vi "TLB Native Dynamic Events ver 0.06.vi"() -> ()   [LabVIEW 2018]
uses:
  Labview Training Phase 2/Enum Controls/States for Action Engine.ctl
  Type def/TLB event states.ctl
  Type def/TLB MHL States.ctl
  <vilib>/Studica/Studica Toolkit/Background/I2C Channel.ctl
  <vilib>/Studica/Studica Toolkit/NavX/NavX.lvlib
  <vilib>/myRIO/Common/Instrument Driver Framework/myRIO v1.0/AI/typedefs/AI Channels Enum.ctl
  <vilib>/myRIO/Common/Instrument Driver Framework/myRIO v1.0/AI/typedefs/AI Channels List.ctl
  <vilib>/Studica/Studica Toolkit/Background/Mxp Selection.ctl
  <vilib>/ptbypt/NI_PtbyPt.lvlib
  Type def/Type def.ctl
  Type def/Motor Control Cluster.ctl
  <vilib>/Studica/Studica Blackhawk/Blackhawk.lvlib
  <vilib>/vision/driver/NI_Vision_Acquisition_Software.lvlib
  <vilib>/userdefined/High Color/IMAQdx.ctl
  <vilib>/vision/driver/IMAQdx.llb/IMAQdx Buffer Number Mode.ctl
  <vilib>/vision/driver/IMAQdx.llb/IMAQdx Acquisition Mode.ctl
panel:
  in  "Camera ENA":bool
  out "Right IR Sensor":dbl
  out "Left IR Sensor":dbl
  out "CM":fxp<+,64,16>
  out "Ultrasonic sensor":dbl format="%0.2f"
  in  "Servo Angle":u8(slide) scale=0.0..180.0
  in  "On/Off":bool
  out "Blackhawk error":errorcluster
  out "Value Read":bool
  out "Image Processing error":errorcluster
  out "Image Out":T1(plugin-control)
  out "element":T2
  out "Action Queue Items":i32
  out "State Logic Queue Items":i32
  out "Action Queues items":string[](array[string])=["Hardware reset", "Software reset", ""]
  out "State logic":T3=enum."Task 2"
  out "Action State":string
  in  "Tasks Selector":string(combo)="Task 2"
  out "Distance":T4
  in  "xTargetSpeed":dbl
  in  "yTargetSpeed":dbl
  in  "wTargetSpeed":dbl
  out "Speed":T5
  out "Yaw":dbl
  out "NavX Info Out":T7
  out "LinearAcceleration":T8
  out "Displacement":T9
  out "YRPHfH":T10
  out "Object detected":bool
  in  "NavX Zero Yaw":bool
  in  "Return to IDLE":bool
  in  "Reset Encoder 0":bool
  in  "Stop Queue":bool
  in  "Start Task":bool
  # "Sensor data"
  # "Blackhawk status"
  # "Camera Status Loop"
  # "TLB FRAMEWORK STATUS"
  # "Test Programme written by Calvin Loke    Dated: 28 Aug 2019\nTest Programme revised by Dr Alex See   Dated 30 Aug 2019\n\nProgramme version:   TLB Native Dynamic Events ver 0.04b.vi"
  # "Sequence of Actions"
  # "Continuous (Repeated)"
  # "System Health Status Update"
  # "Motor Control Loop"
  # "NAVX Control Loop"
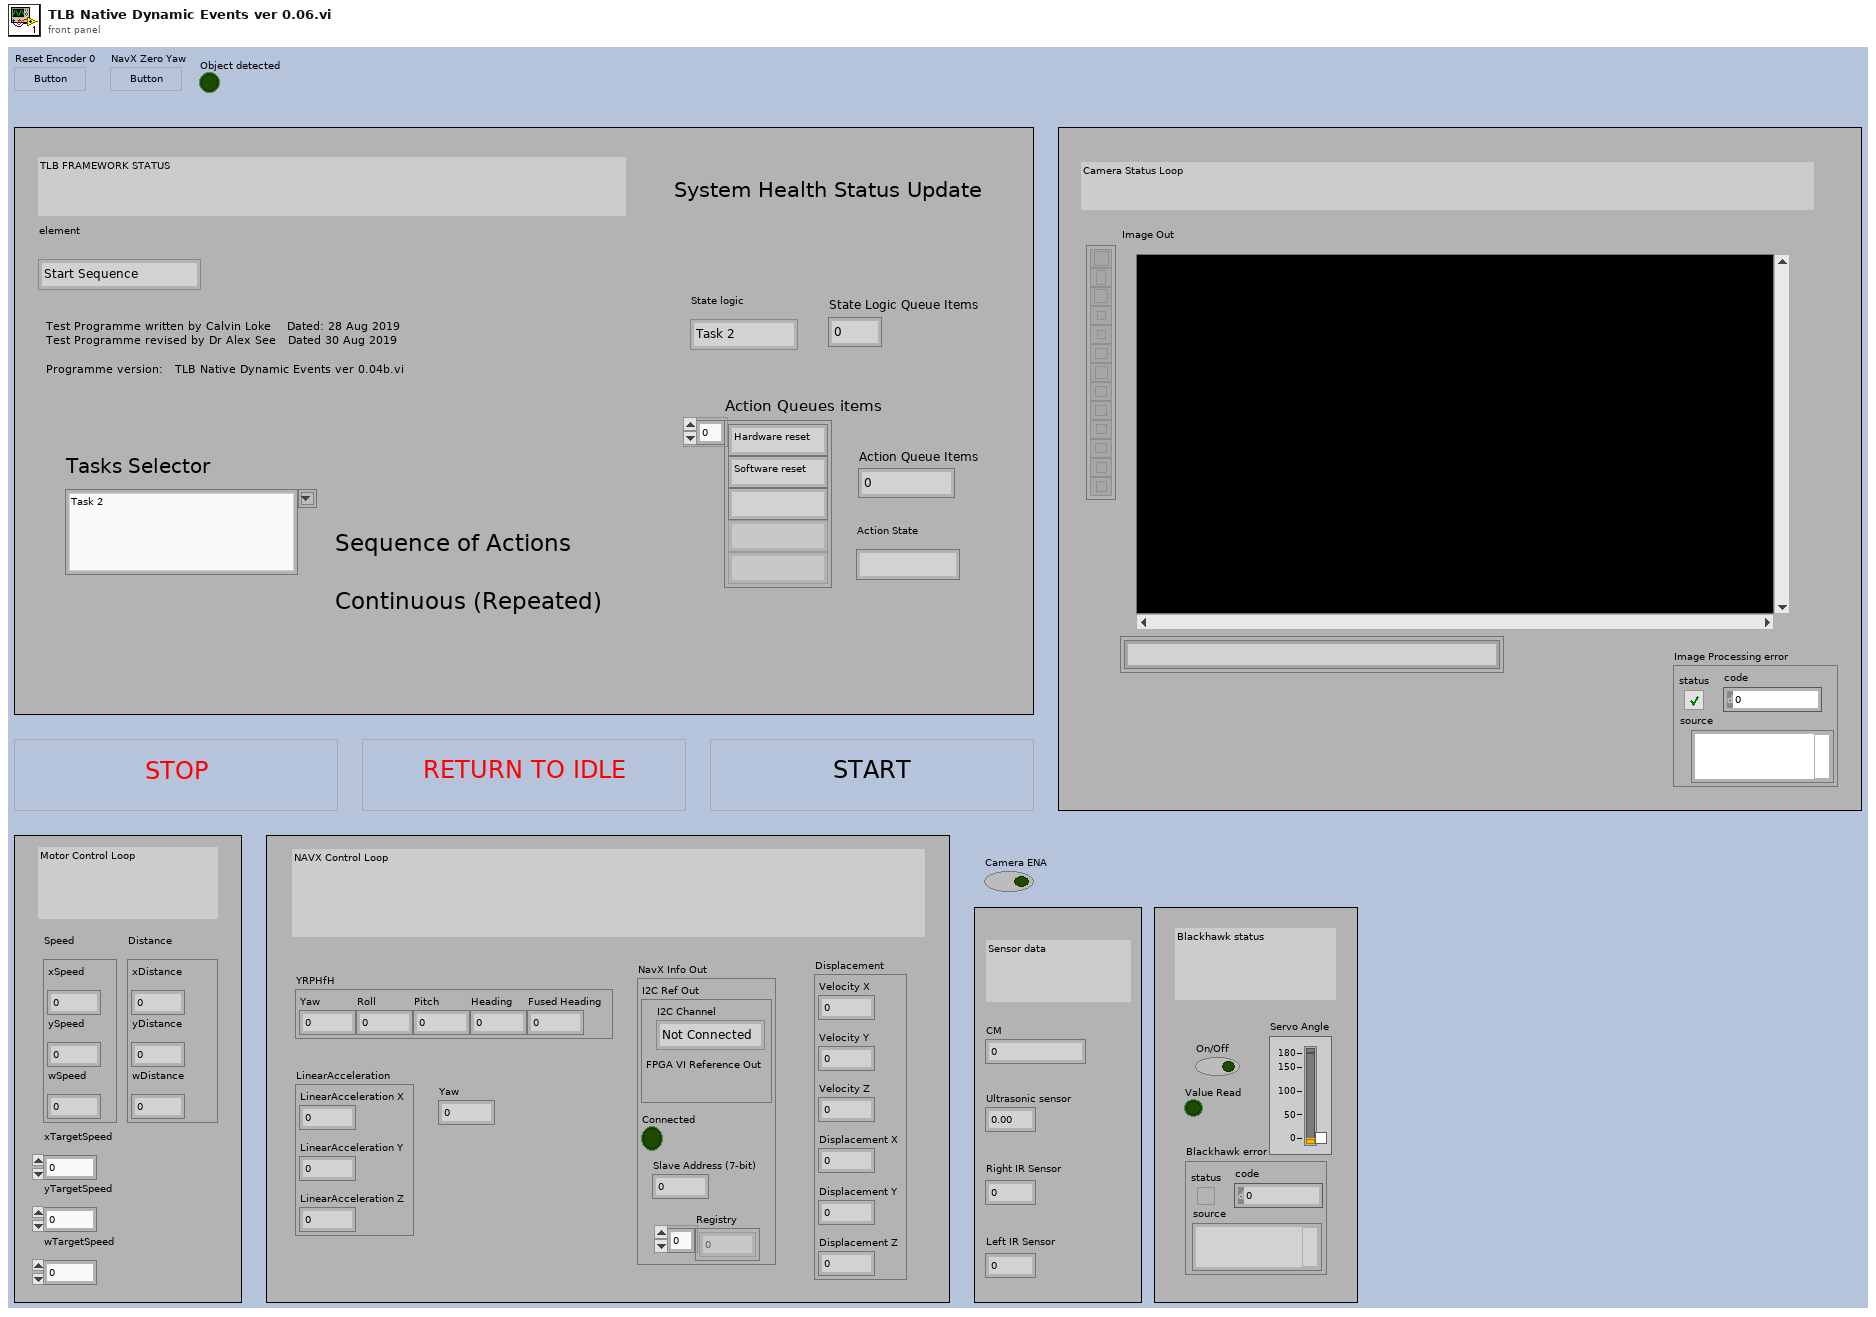
[diagram p1: front panel]
types:
  T1 = typedef "IMAQ Image.ctl" = refnum<image>
  T2 = typedef "TLB event states.ctl" = enum16{"Start Sequence", "Exit", "Start Task 1", "Start Task 2", "Start Task 3", "Start Task 4", "Camera vision", "Wall follow mode", "Idle", "Start Drive Straight"}
  T3 = typedef "TLB MHL States.ctl" = enum16{"None", "Startup", "Idle", "Processing", "Shutdown", "Reset", "Task 1", "Task 2", "Task 3", "Task 4", "Task 4a", "Task 4b", "Task 4c", "Task 4d", "Task 4e", "Task 4f", "Task 4g", "Task 4h", "Acquire image", "Wall follow mode", "Autodrive", "Autodrive a"}
  T4 = cluster{"xDistance":dbl, "yDistance":dbl, "wDistance":dbl}
  T5 = cluster{"xSpeed":dbl, "ySpeed":dbl, "wSpeed":dbl}
  T6 = typedef "I2C Channel.ctl" = enum16{"Not Connected", "A", "B"}
  T7 = cluster{"I2C Ref Out":cluster{"I2C Channel":T6, "FPGA VI Reference Out":refnum<k20>}, "Connected":bool, "Slave Address (7-bit)":u8, "Registry":u8[]}
  T8 = cluster{"LinearAcceleration X":dbl, "LinearAcceleration Y":dbl, "LinearAcceleration Z":dbl}
  T9 = cluster{"Velocity X":dbl, "Velocity Y":dbl, "Velocity Z":dbl, "Displacement X":dbl, "Displacement Y":dbl, "Displacement Z":dbl}
  T10 = cluster{"Yaw":dbl, "Roll":dbl, "Pitch":dbl, "Heading":dbl, "Fused Heading":dbl}
  T11 = typedef "States for Action Engine.ctl" = enum16{"Initialize", "Write", "Read"}
  T12 = typedef "NI_Vision_Acquisition_Software.lvlib/IMAQdx Acquisition Mode.ctl" = enum32{"One Shot", "Continuous"}
  T13 = typedef "IMAQdx.ctl" = refnum<k21>
  T14 = typedef "Motor Control Cluster.ctl" = cluster{"Vx":dbl, "Vy":dbl, "Vw":dbl}
  T15 = typedef "Type def.ctl" = cluster{"Front Ultrasonic Obstruct":bool, "Left Ultrasonic Obstruct":bool, "Right Ultrasonic Obstruct ":bool}
  T16 = typedef "NI_Vision_Acquisition_Software.lvlib/IMAQdx Buffer Number Mode.ctl" = enum32{"Next", "Last", "Buffer Number", "Every", "Last New"}
  T17 = typedef "Mxp Selection.ctl" = enum16{"MXP A", "MXP B"}
  T18 = typedef "TLB event states.ctl" = enum16{"Start Sequence", "Exit", "Start Task 1", "Start Task 2", "Start Task 3", "Start Task 4", "RT Camera tracking", "Wall follow mode", "Idle"}
  T19 = cluster{"I2C Channel":T6, "FPGA VI Reference Out":refnum<k20>}
  T20 = typedef "AI Channels List.ctl" = T21[]
  T21 = typedef "AI Channels Enum.ctl" = enum16{"Not Connected", "AudioIn/Left", "AudioIn/Right", "C/AI0", "C/AI1", "A/AI0", "A/AI1", "A/AI2", "A/AI3", "A/AI4", "A/AI5", "A/AI6", "A/AI7", "B/AI0", "B/AI1", "B/AI2", "B/AI3", "B/AI4", "B/AI5", "B/AI6", "B/AI7", "AI/AI0", "AI/AI1", "AI/AI2", "AI/AI3", "A/AI0 (DIFF)", "A/AI1 (DIFF)", "A/AI2 (DIFF)", "A/AI3 (DIFF)", "B/AI0 (DIFF)", "B/AI1 (DIFF)", "B/AI2 (DIFF)", "B/AI3 (DIFF)"}
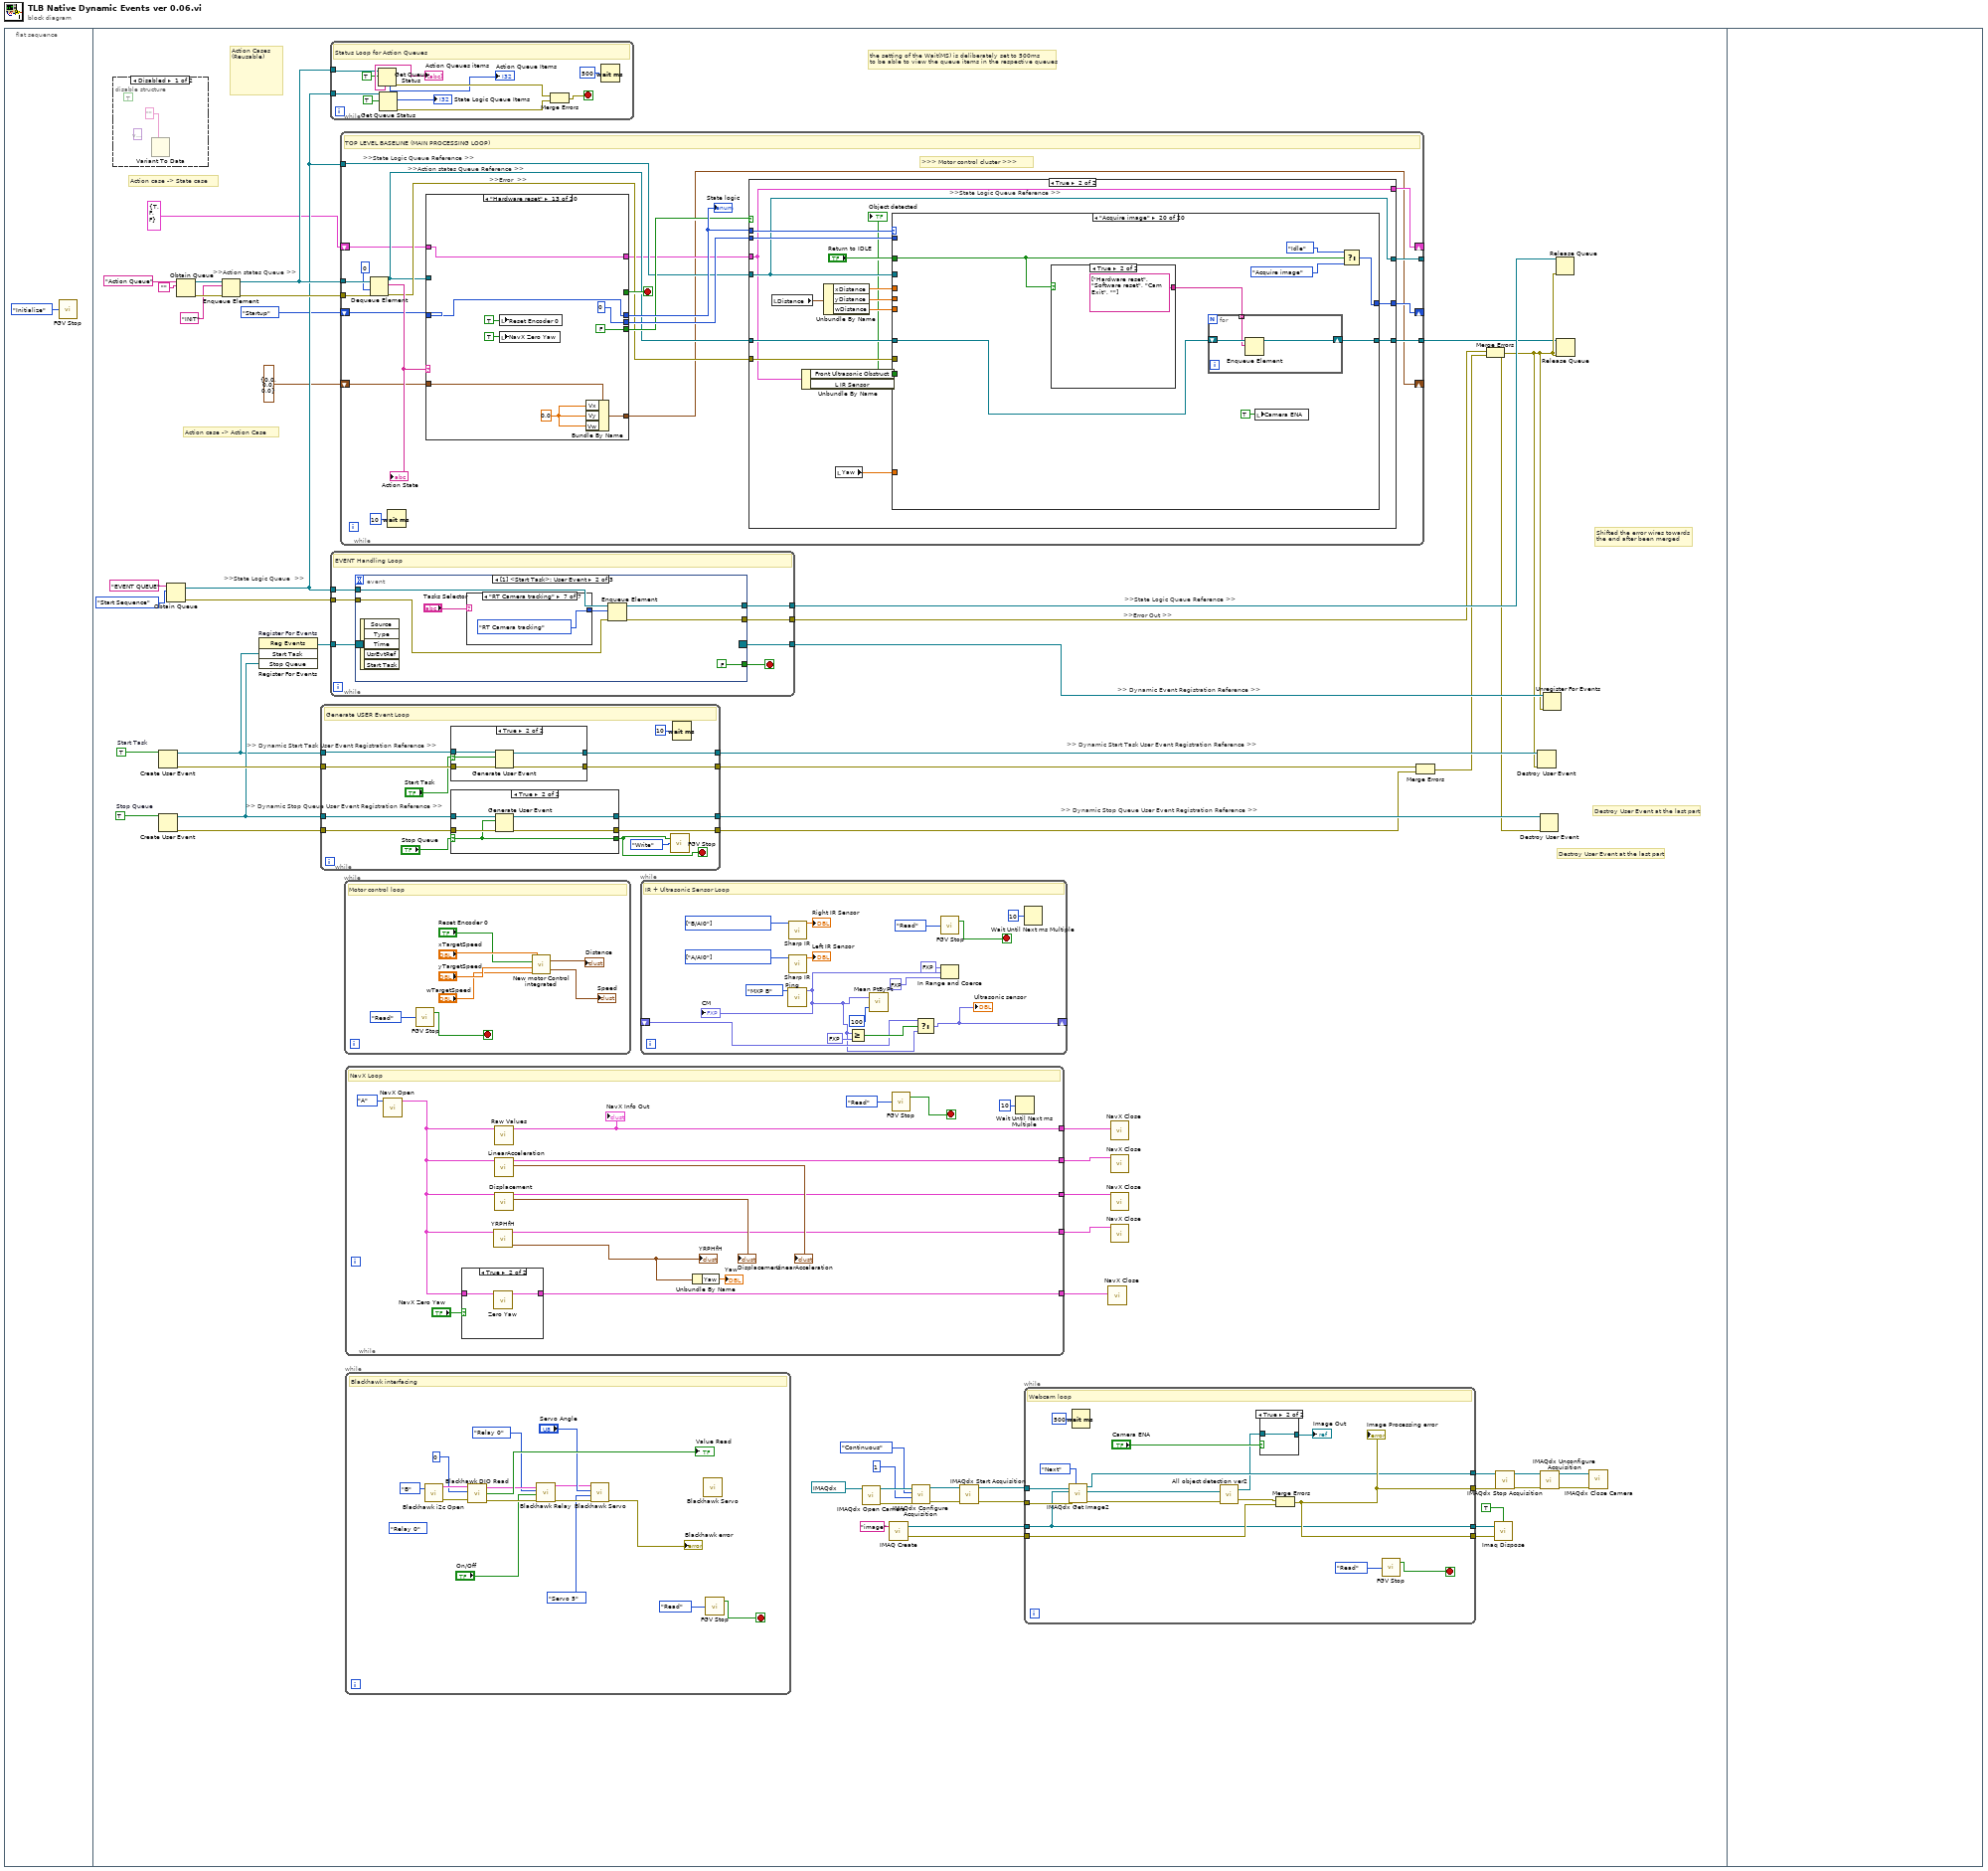
[diagram p0: block diagram]
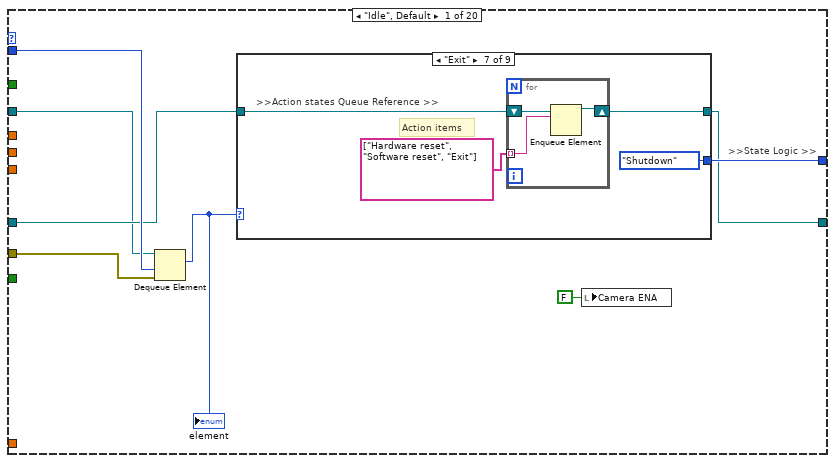
[diagram p6: hidden frame]
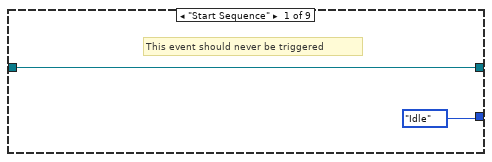
[diagram p7: hidden frame]
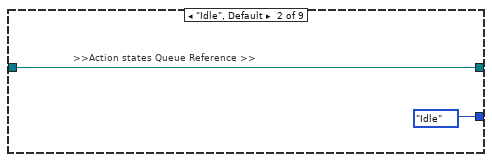
[diagram p8: hidden frame]
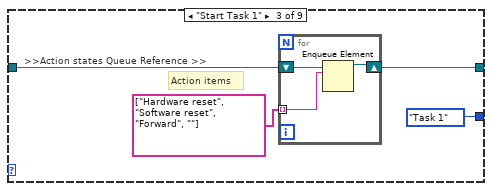
[diagram p9: hidden frame]
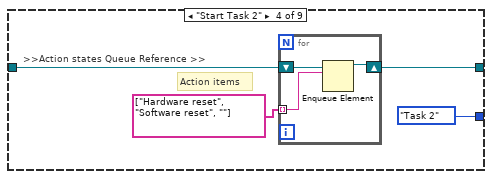
[diagram p10: hidden frame]
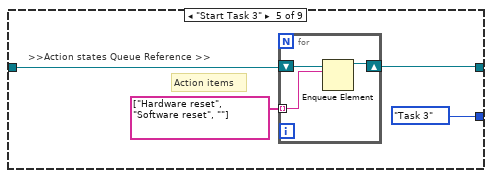
[diagram p11: hidden frame]
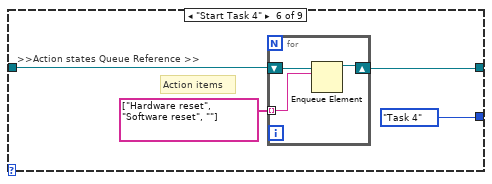
[diagram p12: hidden frame]
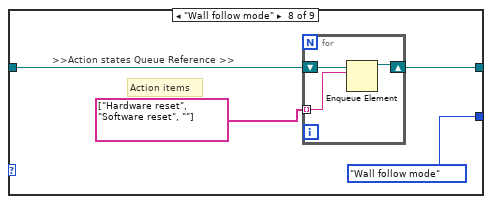
[diagram p13: hidden frame]
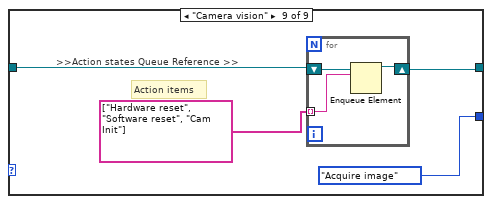
[diagram p14: hidden frame]
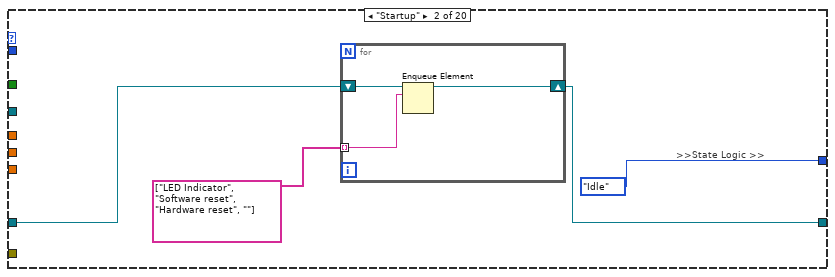
[diagram p15: hidden frame]
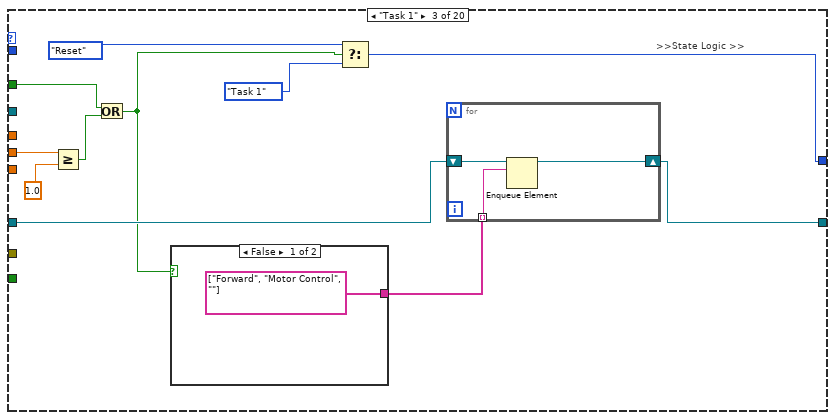
[diagram p16: hidden frame]
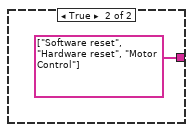
[diagram p17: hidden frame]
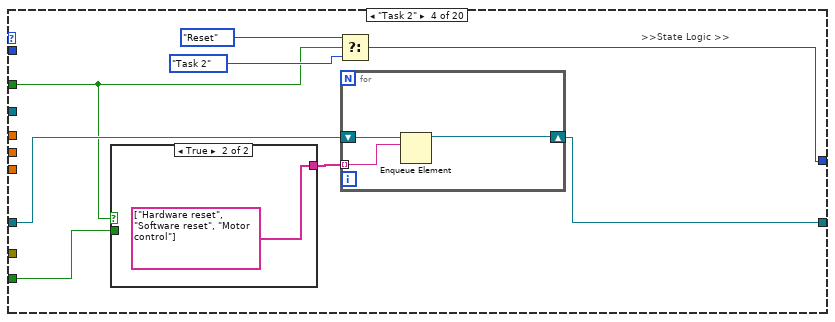
[diagram p18: hidden frame]
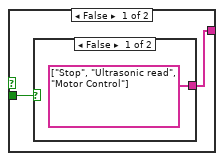
[diagram p19: hidden frame]
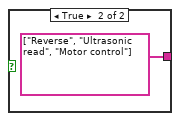
[diagram p20: hidden frame]
diagram:
  n1 = flat-sequence {
    frame #0 {
      n2 = call "FGV Stop.vi"("Init/Read/Write State"=States_for_Action_Engine."Initialize") -> ()  [unwired: 2 in, 2 out]
    }
    frame #1 {
      w58 = TRUE  # Stop Queue
      w57 = TRUE  # Start Task
      # "Action case -> Action Case"
      # "Action case -> State case"
      # "the setting of the Wait(MS) is deliberately set to 500ms\nto be able to view the queue items in the respective queues"
      # "Action Cases\n(Reusable)"
      # ">>Error Out >>"
      # ">> Dynamic Stop Queue User Event Registration Reference >>"
      # ">> Dynamic Start Task User Event Registration Reference >>"
      # ">> Dynamic Stop Queue User Event Registration Reference >>"
      # ">> Dynamic Start Task User Event Registration Reference >>"
      # ">> Dynamic Event Registration Reference >>"
      # ">>Action states Queue >>"
      # ">>State Logic Queue  >>"
      # ">>State Logic Queue Reference >>"
      # "Destroy User Event at the last part"
      # "Destroy User Event at the last part"
      # "Shifted the error wires towards\nthe end after been merged"
      n3 = disable-structure shown="Disabled" {
        frame Disabled {
          (unwired) variant
          (unwired) TRUE
          n4 = Variant To Data(type="") -> ()  [unwired: 2 in, 2 out]
        }
        frame Enabled {
        }
      }
      n5 = Create User Event(user event datatype=w57) -> (user event=w49:refnum<user-event>, error out=w54:errorcluster)  [unwired: 1 in]
      n6 = Create User Event(user event datatype=w58) -> (user event=w50:refnum<user-event>, error out=w53:errorcluster)  [unwired: 1 in]
      n7 = Obtain Queue(name (unnamed)="EVENT QUEUE", element data type=TLB_event_states."Start Sequence" ("Enum")) -> (queue out=w34:refnum<queue>, error out=w40:errorcluster)  [unwired: 3 in, 1 out]
      n8 = Obtain Queue(name (unnamed)="Action Queue", element data type="") -> (queue out=w43:refnum<queue>, error out=w39:errorcluster)  [unwired: 3 in, 1 out]
      n9 = Enqueue Element(queue=w43, element="INIT", error in (no error)=w39) -> (queue out=w35:refnum<queue>, error out=w38:errorcluster)  [unwired: 1 in, 1 out]
      n10 = register-events "Register For Events"(w49, w50) -> (reference out=w48:refnum<event-registration>)  [unwired: 2 in, 1 out]
      n11 = while {
        tunnel: w49 -> [w620]
        tunnel: w50 -> [w619]
        tunnel: [w618] -> w56
        tunnel: [w617] -> w55
        tunnel: w54 -> [w616]
        tunnel: [w615] -> w52
        tunnel: w53 -> [w614]
        tunnel: [w613] -> w51
        stop <- w609 stop-if-true
        # "Generate USER Event Loop"
        n12 = case shown="True" "Start Task" {
          selector: "Start Task" -> [_ w632]
          tunnel: w620 -> [w631 w636]
          tunnel: [w631 w635] -> w617
          tunnel: w616 -> [w630 w634]
          tunnel: [w630 w633] -> w615
          frame False {
          }
          frame True {
            n13 = Generate User Event(user event=w636, event data cluster=w632, error in=w634) -> (user event out=w635:refnum<user-event>, error out=w633:errorcluster)  [unwired: 1 in]
          }
        }
        n14 = case shown="True" "Stop Queue" {
          selector: "Stop Queue" -> [_ w625]
          tunnel: w619 -> [w624 w629]
          tunnel: [w624 w628] -> w618
          tunnel: w614 -> [w623 w627]
          tunnel: [w623 w626] -> w613
          tunnel: [FALSE w625] -> w609
          frame False {
          }
          frame True {
            n15 = Generate User Event(user event=w629, event data cluster=w625, error in=w627) -> (user event out=w628:refnum<user-event>, error out=w626:errorcluster)  [unwired: 1 in]
          }
        }
        n16 = call "FGV Stop.vi"("Init/Read/Write State"=States_for_Action_Engine."Write", "Input Node"=w609) -> ()  [unwired: 1 in, 2 out]
        n17 = Wait (ms)(milliseconds to wait=u32 10) -> ()  [unwired: 1 out]
      }
      n18 = while {
        tunnel: w35 -> [w143]
        tunnel: w34 -> [w140]
        stop <- w137 stop-if-true
        # "Status Loop for Action Queues"
        n19 = Get Queue Status(queue=w143, return elements? (F)=TRUE) -> (error out=w139:errorcluster, # elements in queue=→"Action Queue Items":i32, elements=→"Action Queues items":string[])  [unwired: 1 in, 5 out]
        n20 = Get Queue Status(queue=w140, return elements? (F)=TRUE) -> (# pending remove=→"State Logic Queue Items":i32, error out=w138:errorcluster)  [unwired: 1 in, 6 out]
        n21 = Merge Errors(w139, w138) -> (w137:errorcluster)
        n22 = Wait (ms)(milliseconds to wait=u32 500) -> ()  [unwired: 1 out]
      }
      n23 = while {
        tunnel: w48 -> [w582]
        tunnel: [w581] -> w47
        tunnel: w34 -> [w579]
        tunnel: [w578] -> w46
        tunnel: w40 -> [w577]
        tunnel: [w576] -> w37
        stop <- w580 stop-if-true
        # "EVENT Handling Loop"
        n24 = event shown="[1] <Start Task>: User Event" {
          selector: w582 -> [_ _ _]
          dyn-events: [_ _ _] -> w581
          timeout: _ -> [_ _ _]
          tunnel: [FALSE FALSE w608] -> w580
          tunnel: w579 -> [w587 w594 w606]
          tunnel: [w586 w593 w607] -> w578
          tunnel: w577 -> [w584 w590 w604]
          tunnel: [w583 w589 w603] -> w576
          event Timeout {
            n25 = event-data() -> ()  [unwired: 1 in, 3 out]
            n26 = Enqueue Element(queue=w587, element=TLB_event_states."Idle" ("Enum"), error in (no error)=w584) -> (queue out=w586:refnum<queue>, error out=w583:errorcluster)  [unwired: 1 in, 1 out]
          }
          event User Event {
            n27 = event-data() -> ()  [unwired: 1 in, 5 out]
            n28 = case shown="\"RT Camera tracking\"" "Tasks Selector" {
              tunnel: [TLB_event_states."Idle" ("Enum") TLB_event_states."Start Task 1" ("Enum") TLB_event_states."Start Task 2" ("Enum") TLB_event_states."Start Task 3" ("Enum") TLB_event_states."Start Task 4" ("Enum") TLB_event_states."Wall follow mode" ("Enum") TLB_event_states."RT Camera tracking" ("Enum")] -> w591
              frame Default {
              }
              frame "Task 1" {
              }
              frame "Task 2" {
              }
              frame "Task 3" {
              }
              frame "Task 4" {
              }
              frame "Wall following" {
              }
              frame "RT Camera tracking" {
              }
            }
            n29 = Enqueue Element(queue=w594, element=w591, error in (no error)=w590) -> (queue out=w593:refnum<queue>, error out=w589:errorcluster)  [unwired: 1 in, 1 out]
          }
          event User Event {
            n30 = event-data() -> ("Stop Queue"=w608:bool)  [unwired: 1 in, 4 out]
            n31 = Enqueue Element At Opposite End(queue=w606, element=TLB_event_states."Exit" ("Enum"), error in (no error)=w604) -> (queue out=w607:refnum<queue>, error out=w603:errorcluster)  [unwired: 1 in, 1 out]
          }
        }
      }
      n32 = while {
        tunnel: w34 -> [w154]
        shift-right: [w159] -> _
        shift-left: TLB_MHL_States."Startup" ("Enum") -> [w151]
        tunnel: w35 -> [w164]
        tunnel: w38 -> [w162]
        tunnel: [w161] -> _
        tunnel: [w160] -> w32
        shift-right: [w148] -> _
        shift-left: T15 {"Front Ultrasonic Obstruct"=TRUE, "Left Ultrasonic Obstruct"=FALSE, "Right Ultrasonic Obstruct "=FALSE} -> [w150]
        shift-right: [w146] -> _
        shift-left: T14 {"Vx"=0.0, "Vy"=0.0, "Vw"=0.0} -> [w147]
        stop <- w157 stop-if-true
        # ">>> Motor control cluster >>>"
        # ">>Error  >>"
        # ">>Action states Queue Reference >>"
        # ">>State Logic Queue Reference >>"
        # "TOP LEVEL BASELINE (MAIN PROCESSING LOOP)"
        n33 = Dequeue Element(queue=w164, timeout in ms (-1)=0, error in (no error)=w162) -> (queue out=w152:refnum<queue>, element=w163:string, error out=w153:errorcluster)  [unwired: 1 out]
        "Action State" <- w163
        n34 = Wait (ms)(milliseconds to wait=u32 10) -> ()  [unwired: 1 out]
        n35 = case shown="\"Hardware reset\"" w163 {
          tunnel: [w423 w431 w436 w444 w453 w463 w472 w479 w490 w498 w506 w515 w524 TLB_MHL_States."Shutdown" ("Enum") w539 w543 w557 w563 w566 w575] -> w165
          tunnel: [w422 0 0 0 0 0 0 0 0 0 0 0 0 0 0 0 0 0 0 0] -> w158
          tunnel: [_ _ _ _ _ _ _ _ _ _ _ _ _ TRUE _ _ _ _ _ _] -> w157
          tunnel: [TRUE FALSE FALSE FALSE FALSE FALSE FALSE FALSE FALSE FALSE FALSE FALSE FALSE FALSE FALSE FALSE FALSE FALSE FALSE FALSE] -> w156
          tunnel: w152 -> [_ _ _ _ _ _ _ _ _ _ _ _ _ _ _ _ _ _ _ _]
          tunnel: w151 -> [w423 w431 w436 w444 w453 w463 w472 w479 w490 w498 w506 w515 w524 _ w539 w543 w557 w563 w566 w575]
          tunnel: w150 -> [w420 w428 w433 w440 w449 w458 w467 w476 w485 w494 w507 w512 w519 w526 w538 w546 w558 w564 w565 w571]
          tunnel: [w420 w428 w433 w440 w449 w458 w467 w476 w485 w494 w507 w511 w519 w526 w535 w545 w558 w564 w565 w571] -> w149
          tunnel: w147 -> [w419 w427 w432 w438 w447 w456 w466 w474 w484 w492 w500 w509 w518 w525 w531 w540 w549 w562 w569 w572]
          tunnel: [w419 w427 w432 w439 w448 w457 w465 w475 w483 w493 w500 w509 w516 w525 w531 w540 w550 w562 w569 w572] -> w146
          frame "No action", Default {
            n36 = case shown="\"Startup\", Default" w423 {
              tunnel: [0 100] -> w422
              frame "Startup", Default {
              }
              frame "Idle" {
              }
            }
          }
          frame "Init" {
            # ">>State Logic  >>"
            n37 = local write "Servo Angle"(u8 90 ("Servo Angle")) -> ()
          }
          frame "LED Indicator" {
          }
          frame "Forward" {
            n38 = local write "Reset Encoder 0"(FALSE ("Reset Encoder 0")) -> ()
            n39 = local write "NavX Zero Yaw"(FALSE ("NavX Zero Yaw")) -> ()
            n40 = Bundle By Name(cluster=w438, "Vy"=0.6) -> (w439:T14)
          }
          frame "Reverse" {
            n41 = local write "NavX Zero Yaw"(FALSE ("NavX Zero Yaw")) -> ()
            n42 = local write "Reset Encoder 0"(FALSE ("Reset Encoder 0")) -> ()
            n43 = Bundle By Name(cluster=w447, "Vy"=-0.6) -> (w448:T14)
          }
          frame "Right" {
            n44 = local write "NavX Zero Yaw"(FALSE ("NavX Zero Yaw")) -> ()
            n45 = local write "Reset Encoder 0"(FALSE ("Reset Encoder 0")) -> ()
            n46 = Bundle By Name(cluster=w456, "Vx"=0.6) -> (w457:T14)
          }
          frame "Left" {
            n47 = Bundle By Name(cluster=w466, "Vx"=-0.6) -> (w465:T14)
            n48 = local write "NavX Zero Yaw"(FALSE ("NavX Zero Yaw")) -> ()
            n49 = local write "Reset Encoder 0"(FALSE ("Reset Encoder 0")) -> ()
          }
          frame "Rotate CW" {
            n50 = local write "NavX Zero Yaw"(FALSE ("NavX Zero Yaw")) -> ()
            n51 = local write "Reset Encoder 0"(FALSE ("Reset Encoder 0")) -> ()
            n52 = Bundle By Name(cluster=w474, "Vw"=-0.3) -> (w475:T14)
          }
          frame "Rotate ACW" {
            n53 = local write "Reset Encoder 0"(FALSE ("Reset Encoder 0")) -> ()
            n54 = local write "NavX Zero Yaw"(FALSE ("NavX Zero Yaw")) -> ()
            n55 = Bundle By Name(cluster=w484, "Vw"=0.15) -> (w483:T14)
          }
          frame "Stop" {
            w491 = 0.0
            n56 = local write "NavX Zero Yaw"(FALSE ("NavX Zero Yaw")) -> ()
            n57 = local write "Reset Encoder 0"(FALSE ("Reset Encoder 0")) -> ()
            n58 = Bundle By Name(cluster=w492, "Vx"=w491, "Vy"=w491, "Vw"=w491) -> (w493:T14)
          }
          frame "Motor control" {
            # "Replace with FGV"
            n59 = Unbundle By Name(w500) -> ("Vx"=w503:dbl, "Vy"=w502:dbl, "Vw"=w501:dbl)
            n60 = local write "xTargetSpeed"(w503) -> ()
            n61 = local write "yTargetSpeed"(w502) -> ()
            n62 = local write "wTargetSpeed"(w501) -> ()
          }
          frame "Software reset" {
            w510 = FALSE ("NavX Zero Yaw")
            n63 = local write "NavX Zero Yaw"(w510) -> ()
            n64 = Bundle By Name(cluster=w512, "Front Ultrasonic Obstruct"=w510, "L IR Sensor"=0.0) -> (w511:T15)
          }
          frame "Hardware reset" {
            w517 = 0.0
            n65 = local write "Reset Encoder 0"(TRUE ("Reset Encoder 0")) -> ()
            n66 = local write "NavX Zero Yaw"(TRUE ("NavX Zero Yaw")) -> ()
            n67 = Bundle By Name(cluster=w518, "Vx"=w517, "Vy"=w517, "Vw"=w517) -> (w516:T14)
          }
          frame "Exit" {
          }
          frame "Ultrasonic read" {
            # "Object detection"
            n68 = local read "Ultrasonic sensor"() -> (w534:dbl)
            n69 = Less Or Equal?(x=w534, y=50.0) -> (x <= y?=w532:bool)
            n70 = Bundle By Name(cluster=w538, "Front Ultrasonic Obstruct"=w532) -> (w535:T15)
          }
          frame "IR Sensor Read" {
            n71 = local read "Left IR Sensor"() -> (w544:dbl)
            n72 = Bundle By Name(cluster=w546, "L IR Sensor"=w544) -> (w545:T15)
          }
          frame "Calculate" {
            n73 = Unbundle By Name(w558) -> ("L IR Sensor"=w554:dbl)
            n74 = Subtract(x=w554, y=20.0) -> (x-y=w552:dbl)
            n75 = Multiply(x=w552, y=0.01) -> (x*y=w548:dbl)
            n76 = Bundle By Name(cluster=w549, "Vy"=0.4, "Vw"=w548) -> (w550:T14)
          }
          frame "Cam Init" {
            n77 = local write "Servo Angle"(u8 170 ("Servo Angle")) -> ()
          }
          frame "Cam Acq" {
          }
          frame "Cam Exit" {
            n78 = local write "Servo Angle"(u8 90 ("Servo Angle")) -> ()
          }
        }
        "State logic" <- w165
        n79 = case shown="True" w156 {
          tunnel: w165 -> [w169 w185]
          tunnel: w154 -> [w170 w179]
          tunnel: w152 -> [w168 w184]
          tunnel: [w170 w179] -> w161
          tunnel: [w168 w183] -> w160
          tunnel: [w169 w182] -> w159
          tunnel: w153 -> [_ w181]
          tunnel: w158 -> [_ w180]
          tunnel: w149 -> [w167 w171]
          tunnel: [w167 w171] -> w148
          frame False {
          }
          frame True {
            # ">>State Logic Queue Reference >>"
            n80 = local read "Distance"() -> (w177:T4)
            n81 = Unbundle By Name(w171) -> ("Front Ultrasonic Obstruct"=w172:bool)  [unwired: 1 out]
            "Object detected" <- w172
            n82 = Unbundle By Name(w177) -> ("xDistance"=w174:dbl, "yDistance"=w176:dbl, "wDistance"=w175:dbl)
            n83 = local read "Yaw"() -> (w173:dbl)
            n84 = case shown="\"Acquire image\"" w185 {
              tunnel: w179 -> [w187 _ _ _ _ _ _ _ _ _ _ _ _ _ _ _ _ _ _ _]
              tunnel: w184 -> [w189 w248 w260 w273 w295 w304 w318 w333 w346 w359 w370 w376 w379 w385 w388 w390 w392 w394 w397 w411]
              tunnel: [w188 w247 w259 w274 w294 w305 w317 w332 w345 w358 w369 w376 w378 w385 w388 w390 w392 w394 w398 w410] -> w183
              tunnel: [w192 TLB_MHL_States."Idle" ("Enum") w262 w275 w291 w308 w320 w331 w347 w357 TLB_MHL_States."Idle" ("Enum") TLB_MHL_States."Reset" ("Enum") TLB_MHL_States."Shutdown" ("Enum") TLB_MHL_States."Reset" ("Enum") TLB_MHL_States."Idle" ("Enum") TLB_MHL_States."Idle" ("Enum") TLB_MHL_States."Idle" ("Enum") TLB_MHL_States."Idle" ("Enum") w400 w409] -> w182
              tunnel: w181 -> [w190 _ _ _ _ _ _ _ _ _ _ _ _ _ _ _ _ _ _ _]
              tunnel: w180 -> [w191 _ _ _ _ _ _ _ _ _ _ _ _ _ _ _ _ _ _ _]
              tunnel: "Return to IDLE" -> [_ _ w257 w272 w289 _ _ _ _ _ _ _ _ _ _ _ _ _ w395 w408]
              tunnel: w176 -> [_ _ w256 _ _ _ _ w330 _ _ _ _ _ _ _ _ _ _ _ _]
              tunnel: w175 -> [_ _ _ _ w288 _ _ _ _ _ _ _ _ _ _ _ _ _ _ _]
              tunnel: w174 -> [_ _ _ _ _ _ w314 _ w342 _ _ _ _ _ _ _ _ _ _ _]
              tunnel: w173 -> [_ _ _ _ _ _ _ _ _ _ _ _ _ _ _ _ _ _ _ _]
              tunnel: w172 -> [_ _ _ w270 _ w302 _ _ _ w356 _ _ _ _ _ _ _ _ _ _]
              frame "Idle", Default {
                # ">>State Logic >>"
                n85 = Dequeue Element(queue=w187, timeout in ms (-1)=w191, error in (no error)=w190) -> (element=w193:T2)  [unwired: 3 out]
                "element" <- w193
                n86 = case shown="\"Exit\"" w193 {
                  tunnel: [TLB_MHL_States."Idle" ("Enum") TLB_MHL_States."Idle" ("Enum") TLB_MHL_States."Task 1" ("Enum") TLB_MHL_States."Task 2" ("Enum") TLB_MHL_States."Task 3" ("Enum") TLB_MHL_States."Task 4" ("Enum") TLB_MHL_States."Shutdown" ("Enum") TLB_MHL_States."Wall follow mode" ("Enum") TLB_MHL_States."Acquire image" ("Enum")] -> w192
                  tunnel: [w195 w196 w200 w205 w214 w220 w226 w233 w241] -> w188
                  tunnel: w189 -> [w195 w196 w198 w206 w215 w221 w227 w234 w242]
                  frame "Start Sequence" {
                    # "This event should never be triggered"
                  }
                  frame "Idle", Default {
                    # ">>Action states Queue Reference >>"
                  }
                  frame "Start Task 1" {
                    # ">>Action states Queue Reference >>"
                    # "Action items"
                    n87 = for {
                      shift-right: [w204] -> w200
                      shift-left: w198 -> [w203]
                      tunnel: string[] ["Hardware reset", "Software reset", "Forward", ""] -> [w202] mode=indexing
                      n88 = Enqueue Element(queue=w203, element=w202) -> (queue out=w204:refnum<queue>)  [unwired: 2 in, 2 out]
                    }
                  }
                  frame "Start Task 2" {
                    # ">>Action states Queue Reference >>"
                    # "Action items"
                    n89 = for {
                      shift-right: [w211] -> w205
                      shift-left: w206 -> [w210]
                      tunnel: string[] ["Hardware reset", "Software reset", ""] -> [w209] mode=indexing
                      n90 = Enqueue Element(queue=w210, element=w209) -> (queue out=w211:refnum<queue>)  [unwired: 2 in, 2 out]
                    }
                  }
                  frame "Start Task 3" {
                    # ">>Action states Queue Reference >>"
                    # "Action items"
                    n91 = for {
                      shift-right: [w218] -> w214
                      shift-left: w215 -> [w217]
                      tunnel: string[] ["Hardware reset", "Software reset", ""] -> [w216] mode=indexing
                      n92 = Enqueue Element(queue=w217, element=w216) -> (queue out=w218:refnum<queue>)  [unwired: 2 in, 2 out]
                    }
                  }
                  frame "Start Task 4" {
                    # ">>Action states Queue Reference >>"
                    # "Action items"
                    n93 = for {
                      shift-right: [w225] -> w220
                      shift-left: w221 -> [w224]
                      tunnel: string[] ["Hardware reset", "Software reset", ""] -> [w223] mode=indexing
                      n94 = Enqueue Element(queue=w224, element=w223) -> (queue out=w225:refnum<queue>)  [unwired: 2 in, 2 out]
                    }
                  }
                  frame "Exit" {
                    # ">>Action states Queue Reference >>"
                    # "Action items"
                    n95 = for {
                      shift-right: [w232] -> w226
                      shift-left: w227 -> [w231]
                      tunnel: string[] ["Hardware reset", "Software reset", "Exit"] -> [w230] mode=indexing
                      n96 = Enqueue Element(queue=w231, element=w230) -> (queue out=w232:refnum<queue>)  [unwired: 2 in, 2 out]
                    }
                  }
                  frame "Wall follow mode" {
                    # ">>Action states Queue Reference >>"
                    # "Action items"
                    n97 = for {
                      shift-right: [w239] -> w233
                      shift-left: w234 -> [w238]
                      tunnel: string[] ["Hardware reset", "Software reset", ""] -> [w237] mode=indexing
                      n98 = Enqueue Element(queue=w238, element=w237) -> (queue out=w239:refnum<queue>)  [unwired: 2 in, 2 out]
                    }
                  }
                  frame "Camera vision" {
                    # ">>Action states Queue Reference >>"
                    # "Action items"
                    n99 = for {
                      shift-right: [w246] -> w241
                      shift-left: w242 -> [w245]
                      tunnel: string[] ["Hardware reset", "Software reset", "Cam Init"] -> [w244] mode=indexing
                      n100 = Enqueue Element(queue=w245, element=w244) -> (queue out=w246:refnum<queue>)  [unwired: 2 in, 2 out]
                    }
                  }
                }
                n101 = local write "Camera ENA"(FALSE ("Camera ENA")) -> ()
              }
              frame "Startup" {
                # ">>State Logic >>"
                n102 = for {
                  shift-right: [w252] -> w247
                  shift-left: w248 -> [w253]
                  tunnel: string[] ["LED Indicator", "Software reset", "Hardware reset", ""] -> [w251] mode=indexing
                  n103 = Enqueue Element(queue=w253, element=w251) -> (queue out=w252:refnum<queue>)  [unwired: 2 in, 2 out]
                }
              }
              frame "Task 1" {
                # ">>State Logic >>"
                n104 = Greater Or Equal?(x=w256, y=1.0) -> (x >= y?=w254:bool)
                n105 = Or(x=w257, y=w254) -> (x .or. y?=w258:bool)
                n106 = case shown="False" w258 {
                  tunnel: [string[] ["Forward", "Motor Control", ""] string[] ["Software reset", "Hardware reset", "Motor Control"]] -> w261
                  frame False {
                  }
                  frame True {
                  }
                }
                n107 = Select(t=TLB_MHL_States."Reset" ("Enum"), s=w258, f=TLB_MHL_States."Task 1" ("Enum")) -> (s? t:f=w262:T3)
                n108 = for {
                  shift-right: [w268] -> w259
                  shift-left: w260 -> [w269]
                  tunnel: w261 -> [w267] mode=indexing
                  n109 = Enqueue Element(queue=w269, element=w267) -> (queue out=w268:refnum<queue>)  [unwired: 2 in, 2 out]
                }
              }
              frame "Task 2" {
                # ">>State Logic >>"
                n110 = case shown="True" w272 {
                  tunnel: [w279 string[] ["Hardware reset", "Software reset", "Motor control"]] -> w271
                  tunnel: w270 -> [w278 _]
                  frame False {
                    n111 = case shown="False" w278 {
                      tunnel: [string[] ["Stop", "Ultrasonic read", "Motor Control"] string[] ["Reverse", "Ultrasonic read", "Motor control"]] -> w279
                      frame False {
                      }
                      frame True {
                      }
                    }
                  }
                  frame True {
                  }
                }
                n112 = Select(t=TLB_MHL_States."Reset" ("Enum"), s=w272, f=TLB_MHL_States."Task 2" ("Enum")) -> (s? t:f=w275:T3)
                n113 = for {
                  shift-right: [w284] -> w274
                  shift-left: w273 -> [w285]
                  tunnel: w271 -> [w283] mode=indexing
                  n114 = Enqueue Element(queue=w285, element=w283) -> (queue out=w284:refnum<queue>)  [unwired: 2 in, 2 out]
                }
              }
              frame "Task 3" {
                n115 = Less Or Equal?(x=w288, y=-1.2) -> (x <= y?=w286:bool)
                n116 = Or(x=w286, y=w289) -> (x .or. y?=w290:bool)
                n117 = case shown="True" w290 {
                  tunnel: [string[] ["Rotate CW", "Motor Control"] string[] ["Software reset", "Hardware reset", "Motor Control"]] -> w296
                  frame False {
                  }
                  frame True {
                  }
                }
                n118 = for {
                  shift-right: [w298] -> w294
                  shift-left: w295 -> [w299]
                  tunnel: w296 -> [w297] mode=indexing
                  n119 = Enqueue Element(queue=w299, element=w297) -> (queue out=w298:refnum<queue>)  [unwired: 2 in, 2 out]
                }
                n120 = Select(t=TLB_MHL_States."Reset" ("Enum"), s=w290, f=TLB_MHL_States."Task 3" ("Enum")) -> (s? t:f=w291:T3)
              }
              frame "Task 4" {
                n121 = case shown="False" w302 {
                  tunnel: [string[] ["Forward", "Ultrasonic read", "Motor Control"] string[] ["Stop", "Hardware reset", "Software reset", "Motor Control"]] -> w303
                  frame False {
                  }
                  frame True {
                  }
                }
                n122 = for {
                  shift-right: [w312] -> w305
                  shift-left: w304 -> [w313]
                  tunnel: w303 -> [w311] mode=indexing
                  n123 = Enqueue Element(queue=w313, element=w311) -> (queue out=w312:refnum<queue>)  [unwired: 2 in, 2 out]
                }
                n124 = Select(t=TLB_MHL_States."Task 4a" ("Enum"), s=w302, f=TLB_MHL_States."Task 4" ("Enum")) -> (s? t:f=w308:T3)
              }
              frame "Task 4a" {
                n125 = Greater Or Equal?(x=w314, y=0.5) -> (x >= y?=w316:bool)
                n126 = case shown="True" w316 {
                  tunnel: [string[] ["Right", "Motor Control"] string[] ["Stop", "Hardware reset", "Software reset", "Motor Control"]] -> w319
                  frame False {
                  }
                  frame True {
                  }
                }
                n127 = for {
                  shift-right: [w326] -> w317
                  shift-left: w318 -> [w327]
                  tunnel: w319 -> [w325] mode=indexing
                  n128 = Enqueue Element(queue=w327, element=w325) -> (queue out=w326:refnum<queue>)  [unwired: 2 in, 2 out]
                }
                n129 = Select(t=TLB_MHL_States."Task 4b" ("Enum"), s=w316, f=TLB_MHL_States."Task 4a" ("Enum")) -> (s? t:f=w320:T3)
              }
              frame "Task 4b" {
                n130 = Greater Or Equal?(x=w330, y=0.75) -> (x >= y?=w328:bool)
                n131 = case shown="False" w328 {
                  tunnel: [string[] ["Forward", "Motor control"] string[] ["Stop", "Hardware reset", "Software reset"]] -> w334
                  frame False {
                  }
                  frame True {
                  }
                }
                n132 = for {
                  shift-right: [w340] -> w332
                  shift-left: w333 -> [w341]
                  tunnel: w334 -> [w339] mode=indexing
                  n133 = Enqueue Element(queue=w341, element=w339) -> (queue out=w340:refnum<queue>)  [unwired: 2 in, 2 out]
                }
                n134 = Select(t=TLB_MHL_States."Task 4c" ("Enum"), s=w328, f=TLB_MHL_States."Task 4b" ("Enum")) -> (s? t:f=w331:T3)
              }
              frame "Task 4c" {
                n135 = Less Or Equal?(x=w342, y=-0.65) -> (x <= y?=w343:bool)
                n136 = case shown="False" w343 {
                  tunnel: [string[] ["Left"] string[] ["Stop", "Hardware reset", "Software reset"]] -> w348
                  frame False {
                  }
                  frame True {
                  }
                }
                n137 = for {
                  shift-right: [w354] -> w345
                  shift-left: w346 -> [w355]
                  tunnel: w348 -> [w353] mode=indexing
                  n138 = Enqueue Element(queue=w355, element=w353) -> (queue out=w354:refnum<queue>)  [unwired: 2 in, 2 out]
                }
                n139 = Select(t=TLB_MHL_States."Task 4d" ("Enum"), s=w343, f=TLB_MHL_States."Task 4c" ("Enum")) -> (s? t:f=w347:T3)
              }
              frame "Task 4d" {
                n140 = case shown="False" w356 {
                  tunnel: [string[] ["Forward", "Ultrasonic Read"] string[] ["Stop", "Hardware reset", "Software reset"]] -> w360
                  frame False {
                  }
                  frame True {
                  }
                }
                n141 = for {
                  shift-right: [w366] -> w358
                  shift-left: w359 -> [w367]
                  tunnel: w360 -> [w365] mode=indexing
                  n142 = Enqueue Element(queue=w367, element=w365) -> (queue out=w366:refnum<queue>)  [unwired: 2 in, 2 out]
                }
                n143 = Select(t=TLB_MHL_States."Task 4e" ("Enum"), s=w356, f=TLB_MHL_States."Task 4d" ("Enum")) -> (s? t:f=w357:T3)
              }
              frame "Reset" {
                n144 = for {
                  shift-right: [w374] -> w369
                  shift-left: w370 -> [w375]
                  tunnel: string[] ["Software reset", "Hardware reset", ""] -> [w373] mode=indexing
                  n145 = Enqueue Element(queue=w375, element=w373) -> (queue out=w374:refnum<queue>)  [unwired: 2 in, 2 out]
                }
                n146 = Wait (ms)(milliseconds to wait=u32 250) -> ()  [unwired: 1 out]
              }
              frame "Processing" {
              }
              frame "Shutdown" {
                # ">>State Logic >>"
                n147 = for {
                  shift-right: [w383] -> w378
                  shift-left: w379 -> [w384]
                  tunnel: string[] ["Software reset", "Hardware reset", "Cam Exit", "Exit"] -> [w382] mode=indexing
                  n148 = Enqueue Element(queue=w384, element=w382) -> (queue out=w383:refnum<queue>)  [unwired: 2 in, 2 out]
                }
              }
              frame "None" {
              }
              frame "Task 4e" {
              }
              frame "Task 4f" {
              }
              frame "Task 4g" {
              }
              frame "Task 4h" {
              }
              frame "Wall follow mode" {
                n149 = case shown="True" w395 {
                  tunnel: [string[] ["IR Sensor Read", "Calculate", "Forward", "Motor Control"] string[] ["Hardware reset", "Software reset", "Motor Control"]] -> w396
                  frame False {
                  }
                  frame True {
                  }
                }
                n150 = for {
                  shift-right: [w405] -> w398
                  shift-left: w397 -> [w406]
                  tunnel: w396 -> [w404] mode=indexing
                  n151 = Enqueue Element(queue=w406, element=w404) -> (queue out=w405:refnum<queue>)  [unwired: 2 in, 2 out]
                }
                n152 = Select(t=TLB_MHL_States."Idle" ("Enum"), s=w395, f=TLB_MHL_States."Wall follow mode" ("Enum")) -> (s? t:f=w400:T3)
              }
              frame "Acquire image" {
                n153 = case shown="True" w408 {
                  tunnel: [_ string[] ["Hardware reset", "Software reset", "Cam Exit", ""]] -> w412
                  frame False {
                  }
                  frame True {
                  }
                }
                n154 = for {
                  shift-right: [w417] -> w410
                  shift-left: w411 -> [w418]
                  tunnel: w412 -> [w416] mode=indexing
                  n155 = Enqueue Element(queue=w418, element=w416) -> (queue out=w417:refnum<queue>)  [unwired: 2 in, 2 out]
                }
                n156 = local write "Camera ENA"(TRUE ("Camera ENA")) -> ()
                n157 = Select(t=TLB_MHL_States."Idle" ("Enum"), s=w408, f=TLB_MHL_States."Acquire image" ("Enum")) -> (s? t:f=w409:T3)
              }
            }
          }
        }
      }
      n158 = while {
        stop <- w133 stop-if-true
        # "Motor control loop"
        n159 = call "FGV Stop.vi"("Init/Read/Write State"=States_for_Action_Engine."Read") -> ("Output node"=w133:bool)  [unwired: 2 in, 1 out]
        n160 = call "New motor Control integrated.vi"("wTargetSpeed"="wTargetSpeed", "yTargetSpeed"="yTargetSpeed", "xTargetSpeed"="Reset Encoder 0", "Reset Encoders"="xTargetSpeed") -> ("Speed"=→"Speed":T5, "Distance"=→"Distance":T4)
      }
      n161 = while {
        tunnel: [w103] -> w28
        tunnel: [w100] -> w27
        tunnel: [w99] -> w25
        tunnel: [w98] -> w26
        tunnel: [w95] -> w24
        stop <- w105 stop-if-true
        # "NavX Loop"
        n162 = call <vilib>:"NavX Open.vi"("I2C Channel"=I2C_Channel."A") -> ("NavX Info"=w96:T7)  [unwired: 9 in, 1 out]
        n163 = case shown="True" "NavX Zero Yaw" {
          tunnel: w96 -> [w107 w109]
          tunnel: [w107 w108] -> w95
          frame False {
          }
          frame True {
            n164 = call <vilib>:"Zero Yaw.vi"("NavX Info In"=w109) -> ("NavX Info Out"=w108:T7)  [unwired: 10 in]
          }
        }
        n165 = call <vilib>:"YRPHfH.vi"("NavX Info In"=w96) -> ("YRPHfH"=w93:T10, "NavX Info Out"=w99:T7)  [unwired: 3 in]
        "YRPHfH" <- w93
        n166 = call <vilib>:"Raw Values.vi"("NavX Info In"=w96) -> ("NavX Info Out"=w103:T7)  [unwired: 8 in, 1 out]
        "NavX Info Out" <- w103
        n167 = call <vilib>:"LinearAcceleration.vi"("NavX Info In"=w96) -> ("LinearAcceleration"=→"LinearAcceleration":T8, "NavX Info Out"=w100:T7)  [unwired: 9 in]
        n168 = call <vilib>:"Displacement.vi"("NavX Info In"=w96) -> ("Displacement"=→"Displacement":T9, "NavX Info Out"=w98:T7)  [unwired: 9 in]
        n169 = Unbundle By Name(w93) -> ("Yaw"=→"Yaw":dbl)
        n170 = call "FGV Stop.vi"("Init/Read/Write State"=States_for_Action_Engine."Read") -> ("Output node"=w105:bool)  [unwired: 2 in, 1 out]
        n171 = Wait Until Next ms Multiple(millisecond multiple=u32 10) -> ()  [unwired: 1 out]
      }
      n172 = while {
        stop <- w85 stop-if-true
        (unwired) enum8{"Relay 0", "Relay 1", "Relay 2"}."Relay 0" ("Relay")
        # "Blackhawk interfacing"
        n173 = call <vilib>:"Blackhawk i2c Open.vi"("I2C Channel"=I2C_Channel."B") -> ("I2C Ref Out"=w91:T19, "error out"=w90:errorcluster)  [unwired: 2 in]
        n174 = call <vilib>:"Blackhawk DIO Read.vi"("I2C Ref In"=w91, "PIN"=u8 0, "error in (no error)"=w90) -> ("I2C Ref Out"=w83:T19, "Value Read"=→"Value Read":bool, "error out"=w84:errorcluster)  [unwired: 3 in]
        n175 = call <vilib>:"Blackhawk Relay.vi"("error in (no error)"=w84, "On/Off"="On/Off", "Relay"=enum8{"Relay 0", "Relay 1", "Relay 2"}."Relay 0", "I2C Ref In"=w83) -> ("error out"=w80:errorcluster, "I2C Ref Out"=w76:T19)  [unwired: 6 in]
        n176 = call <vilib>:"Blackhawk Servo.vi"("error in (no error)"=w80, "Servo Select"=enum16{"Servo 5", "Servo 6"}."Servo 5", "Servo Angle"="Servo Angle", "I2C Ref In"=w76) -> ("error out"=→"Blackhawk error":errorcluster)  [unwired: 6 in, 1 out]
        n177 = call <vilib>:"Blackhawk Servo.vi"() -> ()  [unwired: 10 in, 2 out]
        n178 = call "FGV Stop.vi"("Init/Read/Write State"=States_for_Action_Engine."Read") -> ("Output node"=w85:bool)  [unwired: 2 in, 1 out]
      }
      n179 = while {
        shift-right: [w114] -> _
        shift-left: _ -> [w115]
        stop <- w120 stop-if-true
        w125 = T20 [enum."A/AI0"] items=["Not Connected", "AudioIn/Left", "AudioIn/Right", "C/AI0", "C/AI1", "A/AI0", "A/AI1", "A/AI2", "A/AI3", "A/AI4", "A/AI5", "A/AI6", "A/AI7", "B/AI0", "B/AI1", "B/AI2", "B/AI3", "B/AI4", "B/AI5", "B/AI6", "B/AI7", "AI/AI0", "AI/AI1", "AI/AI2", "AI/AI3", "A/AI0 (DIFF)", "A/AI1 (DIFF)", "A/AI2 (DIFF)", "A/AI3 (DIFF)", "B/AI0 (DIFF)", "B/AI1 (DIFF)", "B/AI2 (DIFF)", "B/AI3 (DIFF)"] ("AI Channel")
        w126 = T20 [enum."B/AI0"] items=["Not Connected", "AudioIn/Left", "AudioIn/Right", "C/AI0", "C/AI1", "A/AI0", "A/AI1", "A/AI2", "A/AI3", "A/AI4", "A/AI5", "A/AI6", "A/AI7", "B/AI0", "B/AI1", "B/AI2", "B/AI3", "B/AI4", "B/AI5", "B/AI6", "B/AI7", "AI/AI0", "AI/AI1", "AI/AI2", "AI/AI3", "A/AI0 (DIFF)", "A/AI1 (DIFF)", "A/AI2 (DIFF)", "A/AI3 (DIFF)", "B/AI0 (DIFF)", "B/AI1 (DIFF)", "B/AI2 (DIFF)", "B/AI3 (DIFF)"] ("AI Channel")
        # "IR + Ultrasonic Sensor Loop"
        n180 = call <vilib>:"Ping.vi"("Mxp Side"=Mxp_Selection."MXP B") -> ("CM"=w113:fxp<+,64,16>)  [unwired: 8 in, 2 out]
        "CM" <- w113
        n181 = call <vilib>:"Sharp IR.vi"("AI Channel"=w126) -> ("Sharp IR Distance"=→"Right IR Sensor":dbl)  [unwired: 8 in, 2 out]
        n182 = call <vilib>:"Sharp IR.vi"("AI Channel"=w125) -> ("Sharp IR Distance"=→"Left IR Sensor":dbl)  [unwired: 8 in, 2 out]
        n183 = Greater Or Equal?(x=w113, y=fxp<+,64,16> 299.0) -> (x >= y?=w116:bool)
        n184 = call <vilib>:"Mean PtByPt.vi"("x"=w113, "sample length"=100) -> ()  [unwired: 2 in, 2 out]
        n185 = Select(t=w115, s=w116, f=w113) -> (s? t:f=w114:fxp<+,64,16>)
        "Ultrasonic sensor" <- w114
        n186 = call "FGV Stop.vi"("Init/Read/Write State"=States_for_Action_Engine."Read") -> ("Output node"=w120:bool)  [unwired: 2 in, 1 out]
        n187 = In Range and Coerce(upper limit=fxp<+,64,16> 250.0, x=w113, lower limit=fxp<+,64,16> 0.0 ("CM")) -> ()  [unwired: 2 out]
        n188 = Wait Until Next ms Multiple(millisecond multiple=u32 10) -> ()  [unwired: 1 out]
      }
      n189 = call <vilib>:"IMAQdx Open Camera.vi"("Session In"=T13 "cam1") -> ("error out"=w6:errorcluster, "Session Out"=w8:T13)  [unwired: 9 in]
      n190 = call "IMAQ Create"("Image Name"="image") -> ("New Image"=w21:T1, "error out"=w20:errorcluster)  [unwired: 4 in]
      n191 = call <vilib>:"IMAQdx Configure Acquisition.vi"("error in"=w6, "Number of Buffers"=u32 1, "Continuous?"=IMAQdx_Acquisition_Mode."Continuous", "Session In"=w8) -> ("error out"=w5:errorcluster, "Session Out"=w7:T13)  [unwired: 6 in]
      n192 = call <vilib>:"IMAQdx Start Acquisition.vi"("error in"=w5, "Session In"=w7) -> ("error out"=w15:errorcluster, "Session Out"=w16:T13)  [unwired: 8 in]
      n193 = while {
        tunnel: w21 -> [w67]
        tunnel: w20 -> [w71]
        tunnel: [w67] -> w19
        tunnel: [w70] -> w18
        tunnel: [w70] -> w10
        tunnel: w16 -> [w69]
        tunnel: w15 -> [w68]
        tunnel: [w65] -> w9
        stop <- w73 stop-if-true
        # "Webcam loop"
        n194 = call <vilib>:"IMAQdx Get Image2.vi"("Buffer Number Mode (Next)"=IMAQdx_Buffer_Number_Mode."Next", "error in"=w68, "Image In"=w67, "Session In"=w69) -> ("error out"=w62:errorcluster, "Image Out"=w63:T1, "Session Out"=w65:T13)  [unwired: 4 in, 1 out]
        n195 = Wait (ms)(milliseconds to wait=u32 500) -> ()  [unwired: 1 out]
        n196 = call "All object detection ver2.vi"("error in"=w62, "Image In"=w63) -> ("error out"=w64:errorcluster, "Image Out"=w60:T1)
        n197 = case shown="True" "Camera ENA" {
          tunnel: [_ w75] -> w59
          tunnel: w60 -> [_ w75]
          frame False {
          }
          frame True {
          }
        }
        "Image Out" <- w59
        n198 = Merge Errors(w64, w71) -> (w70:errorcluster)
        "Image Processing error" <- w70
        n199 = call "FGV Stop.vi"("Init/Read/Write State"=States_for_Action_Engine."Read") -> ("Output node"=w73:bool)  [unwired: 2 in, 1 out]
      }
      n200 = call <vilib>:"NavX Close.vi"("NavX Info In"=w24) -> ()  [unwired: 10 in, 1 out]
      n201 = call <vilib>:"NavX Close.vi"("NavX Info In"=w28) -> ()  [unwired: 10 in, 1 out]
      n202 = call <vilib>:"NavX Close.vi"("NavX Info In"=w27) -> ()  [unwired: 10 in, 1 out]
      n203 = call <vilib>:"NavX Close.vi"("NavX Info In"=w26) -> ()  [unwired: 10 in, 1 out]
      n204 = call <vilib>:"NavX Close.vi"("NavX Info In"=w25) -> ()  [unwired: 10 in, 1 out]
      n205 = Merge Errors "Merge Errors"(w52, w51) -> (w31:errorcluster)
      n206 = Merge Errors(w37, w31) -> (w33:errorcluster)
      n207 = call "Imaq Dispose"("All Images? (No)"=TRUE, "Image"=w19, "error in (no error)"=w18) -> ()  [unwired: 3 in, 1 out]
      n208 = call <vilib>:"IMAQdx Stop Acquisition.vi"("error in"=w10, "Session In"=w9) -> ("error out"=w13:errorcluster, "Session Out"=w14:T13)  [unwired: 8 in]
      n209 = Destroy User Event(user event=w55, error in=w33) -> ()  [unwired: 1 out]
      n210 = Destroy User Event(user event=w56, error in=w33) -> ()  [unwired: 1 out]
      n211 = call <vilib>:"IMAQdx Unconfigure Acquisition.vi"("error in"=w13, "Session In"=w14) -> ("error out"=w11:errorcluster, "Session Out"=w12:T13)  [unwired: 8 in]
      n212 = Unregister For Events(event registration refnum=w47, error in=w33) -> ()  [unwired: 1 out]
      n213 = Release Queue(queue=w46, error in (no error)=w33) -> ()  [unwired: 1 in, 3 out]
      n214 = Release Queue(queue=w32, error in (no error)=w33) -> ()  [unwired: 1 in, 3 out]
      n215 = call <vilib>:"IMAQdx Close Camera.vi"("error in"=w11, "Session In"=w12) -> ()  [unwired: 9 in, 1 out]
    }
    frame #2 {
    }
  }
